vi "ReadSyringeConfiguration.vi"(0 "object in":refnum<class "CetoniPump.lvclass">, 5 "error in (no error)":errorcluster) -> (14 "object out":refnum<class "CetoniPump.lvclass">, 16 "COnfigured Syringes":T1(array[cluster]), 19 "error out":errorcluster)   [LabVIEW 2021, in "CetoniPump.lvclass"]
uses:
  CetoniPump.lvclass
  CetoniPump.lvclass/CetoniPump.ctl
  CETONI_SDK/lib/labview/labbCAN_Pump_API/labbCAN_Pump_API.lvlib
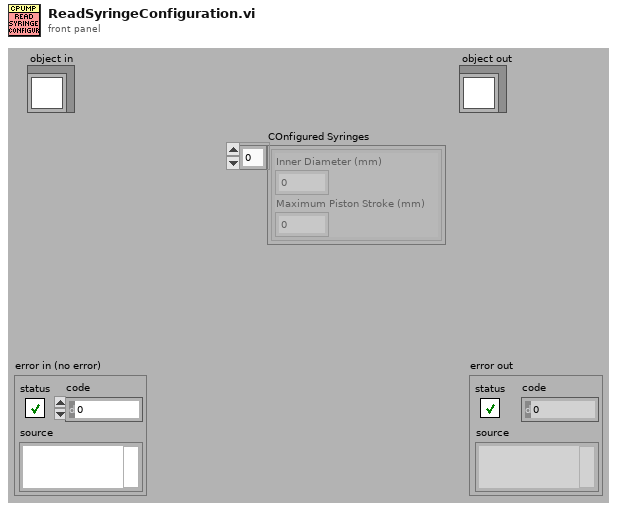
[diagram p1: front panel]
types:
  T1 = cluster{"Inner Diameter (mm)":dbl, "Maximum Piston Stroke (mm)":dbl}[]
  T2 = cluster{"Inner Diameter (mm)":dbl, "Maximum Piston Stroke (mm)":dbl}
  T3 = cluster{"Pump Handle":i64, "Pump Name":string, "Maximum Volume":dbl, "Maximum Flow Rate":dbl, "Flow Rate":dbl, "Target Level":dbl}[]
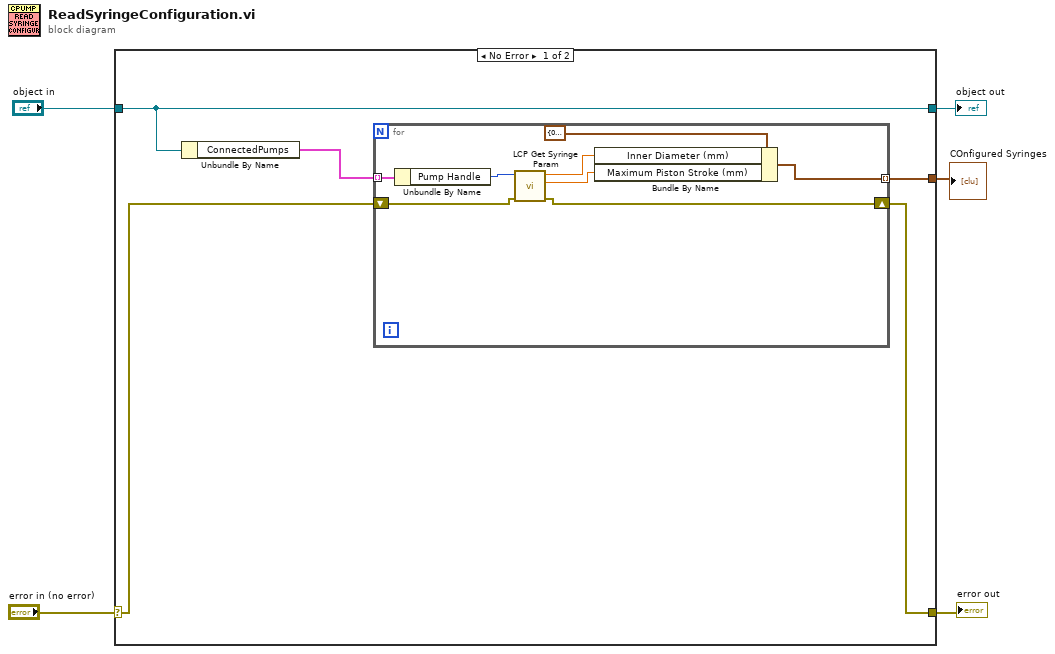
[diagram p0: block diagram]
diagram:
  n1 = case shown="No Error" "error in (no error)" {
    selector: "error in (no error)" -> [w8 w20]
    tunnel: [w7 w20] -> w4
    tunnel: [w10 w19] -> w2
    tunnel: "object in" -> [w10 w19]
    tunnel: [w6 _] -> w1
    frame No Error {
      n2 = Unbundle By Name(w10) -> ("ConnectedPumps"=w9:T3)
      n3 = for {
        tunnel: w9 -> [w18] mode=indexing
        shift-right: [w15] -> w7
        shift-left: w8 -> [w16]
        tunnel: [w14] -> w6 mode=indexing
        n4 = Unbundle By Name(w18) -> ("Pump Handle"=w17:i64)
        n5 = call "LCP Get Syringe Param.vi"("error in (no error)"=w16, "Pump Handle"=w17) -> ("error out"=w15:errorcluster, "Maximum Piston Stroke (mm)"=w11:dbl, "Inner Diameter (mm)"=w12:dbl)  [unwired: 7 in]
        n6 = Bundle By Name(cluster=T2 {"Inner Diameter (mm)"=0.0, "Maximum Piston Stroke (mm)"=0.0} ("COnfigured Syringes 2"), "Inner Diameter (mm)"=w12, "Maximum Piston Stroke (mm)"=w11) -> (w14:T2)
      }
    }
    frame Error {
    }
  }
  "error out" <- w4
  "object out" <- w2
  "COnfigured Syringes" <- w1
